vi "Create Buffer.vi"(6 "Buffer Style (1: Standard)":i32(ring)=1 items=["Compact", "Standard", "Full", "Writable", "Full Writable"], 7 "Fill Type (0: Continuous)":i32(ring) items=["Continuous", "Once"], 8 "error in (no error)":errorcluster, 9 "Buffer Size (10)":u32=10, 10 "Buffer Name (\"\")":string, 11 "VISA resource name":refnum<visa-resource-name>) -> (0 "error out":errorcluster, 3 "VISA resource name out":refnum<visa-resource-name>)   [LabVIEW 2023, in "Keithley DMM6500 DAQ6500 Series.lvlib"]
doc: "Creates a buffer for trigger and scan, and corresponding settings."
uses:
  <instrlib>/Keithley DMM6500 DAQ6500 Series/Keithley DMM6500 DAQ6500 Series.lvlib
  <vilib>/Utility/error.llb/Trim Whitespace One-Sided.vi
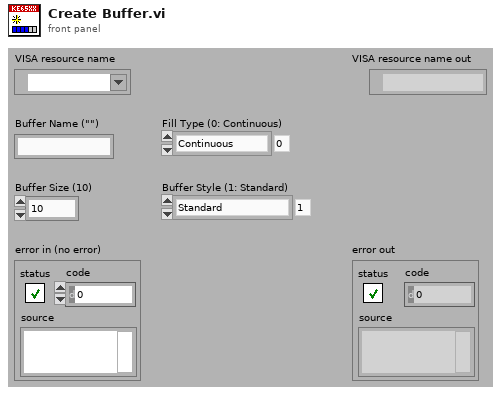
[diagram p1: front panel]
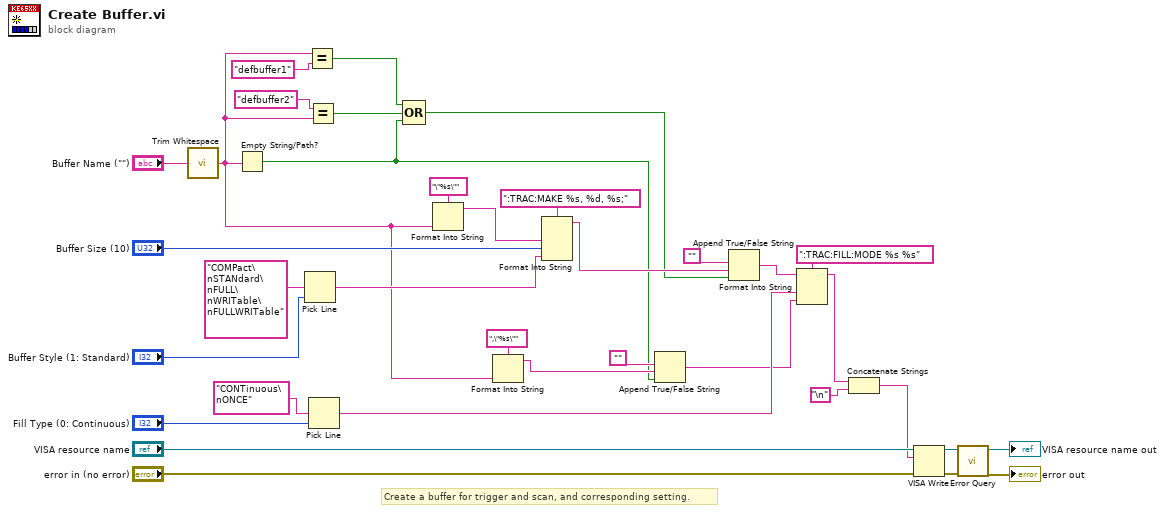
[diagram p0: block diagram]
diagram:
  # "Create a buffer for trigger and scan, and corresponding setting."
  n1 = call <vilib>:"Trim Whitespace.vi"("string"="Buffer Name (\"\")") -> ("trimmed string"=w4:string)  [unwired: 1 in]
  n2 = Empty String/Path?(string/path=w4) -> (empty?=w3:bool)
  n3 = Pick Line(multi-line string="COMPact\nSTANdard\nFULL\nWRITable\nFULLWRITable", line index="Buffer Style (1: Standard)") -> (output string=w25:string)  [unwired: 1 in]
  n4 = Equal?(x=w4, y="defbuffer1") -> (x = y?=w7:bool)
  n5 = Equal?(x="defbuffer2", y=w4) -> (x = y?=w6:bool)
  n6 = Pick Line(multi-line string="CONTinuous\nONCE", line index="Fill Type (0: Continuous)") -> (output string=w22:string)  [unwired: 1 in]
  n7 = Compound Arithmetic op=OR(w7, w6, w3) -> (w5:bool)
  n8 = Format Into String(format string="\"%s\"", w4) -> (resulting string=w11:string)  [unwired: 2 in, 1 out]
  n9 = Format Into String(format string=",\"%s\"", w4) -> (resulting string=w8:string)  [unwired: 2 in, 1 out]
  n10 = Format Into String(format string=":TRAC:MAKE %s, %d, %s;", w11, "Buffer Size (10)", w25) -> (resulting string=w15:string)  [unwired: 2 in, 1 out]
  n11 = Append True/False String(1:w3, 2:w8, 3:"") -> (0:w9:string)  [unwired: 1 in]
  n12 = Append True/False String(1:w5, 2:w15, 3:"") -> (0:w17:string)  [unwired: 1 in]
  n13 = Format Into String(format string=":TRAC:FILL:MODE %s %s", initial string=w17, w22, w9) -> (resulting string=w21:string)  [unwired: 1 in, 1 out]
  n14 = Concatenate Strings(w21, "\n") -> (w20:string)
  n15 = VISA Write(VISA resource name="VISA resource name", write buffer=w20, error in (no error)="error in (no error)") -> (VISA resource name out=w31:refnum<visa-resource-name>, error out=w30:errorcluster)  [unwired: 1 out]
  n16 = call <instrlib>:"Error Query.vi"("error in (no error)"=w30, "VISA resource name"=w31) -> ("error out"=→"error out":errorcluster, "VISA resource name out"=→"VISA resource name out":refnum<visa-resource-name>)  [unwired: 6 in, 2 out]
